vi "Select Symbol.vi"(9 "Name":string, 11 "Symbol":T1) -> (3 "Symbol ID":string)   [LabVIEW 2020, in "VI Properties Editor.lvlib" / "Project Tree Map.lvclass"]
doc: "Selects the symbol ID to use, based on the contents of <B>Symbol</B> and <B>Name</B>."
uses:
  Project Tree Map.lvclass
  <vilib>/picture/picture.llb/imagedata.ctl
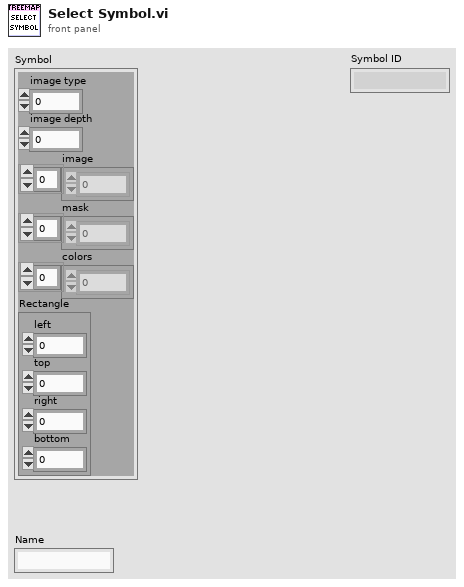
[diagram p1: front panel]
types:
  T1 = typedef "imagedata.ctl" = cluster{"image type":i32, "image depth":i32, "image":u8[], "mask":u8[], "colors":u32[], "Rectangle":cluster{"left":i16, "top":i16, "right":i16, "bottom":i16}}
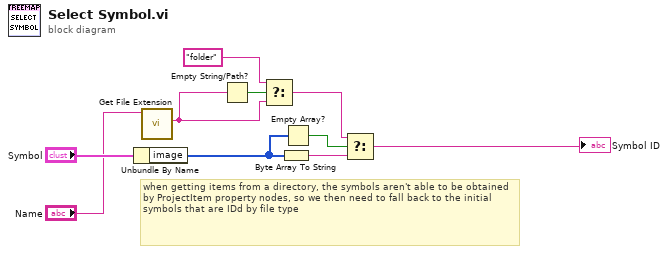
[diagram p0: block diagram]
diagram:
  # "when getting items from a directory, the symbols aren't able to be obtained by ProjectItem property nodes, so we then need to fall back to the initial symbols that are IDd by file type"
  n1 = Unbundle By Name("Symbol") -> ("image"=w8:u8[])
  n2 = call "Get File Extension.vi"("Filename"="Name") -> ("Lowercase Extension"=w3:string)  [unwired: 9 in, 1 out]
  n3 = Empty String/Path?(string/path=w3) -> (empty?=w4:bool)
  n4 = Select(t="folder", s=w4, f=w3) -> (s? t:f=w1:string)
  n5 = Byte Array To String(unsigned byte array=w8) -> (string=w6:string)
  n6 = Empty Array?(array=w8) -> (empty?=w7:bool)
  n7 = Select(t=w1, s=w7, f=w6) -> (s? t:f=→"Symbol ID":string)
